vi "Write Repeat.vi"(8 "error in (no error)":errorcluster, 10 "Repeat":i32, 11 "Action Step in":refnum<class "Action Step.lvclass">) -> (0 "error out":errorcluster, 3 "Action Step out":refnum<class "Action Step.lvclass">)   [LabVIEW 2020, in "MacroAssert.lvlib" / "Action Step.lvclass"]
uses:
  Action Step.lvclass
  Action Step.lvclass/Action Step.ctl
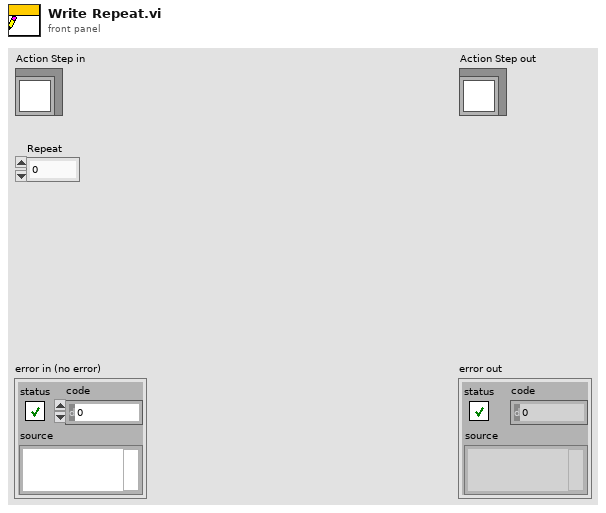
[diagram p1: front panel]
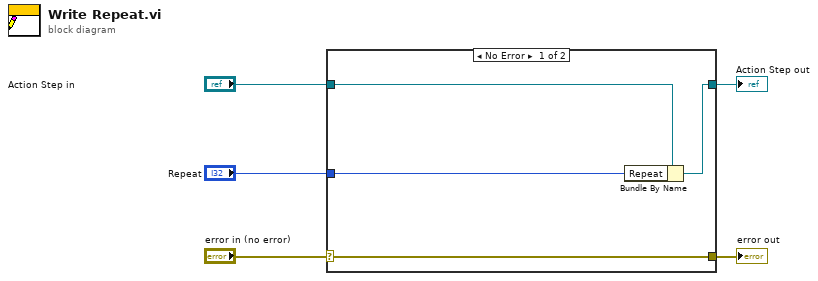
[diagram p0: block diagram]
diagram:
  n1 = case shown="No Error" "error in (no error)" {
    selector: "error in (no error)" -> [w9 w10]
    tunnel: [w9 w10] -> w4
    tunnel: [w7 w11] -> w2
    tunnel: "Action Step in" -> [w8 w11]
    tunnel: "Repeat" -> [w6 _]
    frame No Error {
      n2 = Bundle By Name(cluster=w8, "Repeat"=w6) -> (w7:refnum<class "Action Step.lvclass">)
    }
    frame Error {
    }
  }
  "error out" <- w4
  "Action Step out" <- w2
